vi "ACal-Update Probe Tube Parameters.vi"(0 "Params in":T1) -> (4 "Params out":T1)   [LabVIEW 2020]
uses:
  Type Defs/ACal-Probe Tube Parameters.ctl
  epl-vi-lib/Utility VIs/Type Defs/Left-Right ring.ctl
  Type Defs/Cal Stimulus.ctl
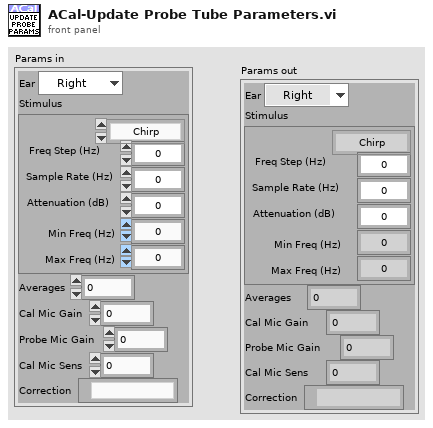
[diagram p1: front panel]
types:
  T1 = typedef "ACal-Probe Tube Parameters.ctl" = cluster{"Ear":T2, "Stimulus":T3, "Averages":i32, "Cal Mic Gain":dbl, "Probe Mic Gain":dbl, "Cal Mic Sens":dbl, "Correction":path}
  T2 = typedef "Left-Right ring.ctl" = enum16{"Right", "Left"}
  T3 = typedef "Cal Stimulus.ctl" = cluster{"Min Freq (Hz)":dbl, "Max Freq (Hz)":dbl, "Freq Step (Hz)":dbl, "Waveform":enum16{"Chirp", "Weighted"}, "Attenuation (dB)":dbl, "Sample Rate (Hz)":dbl}
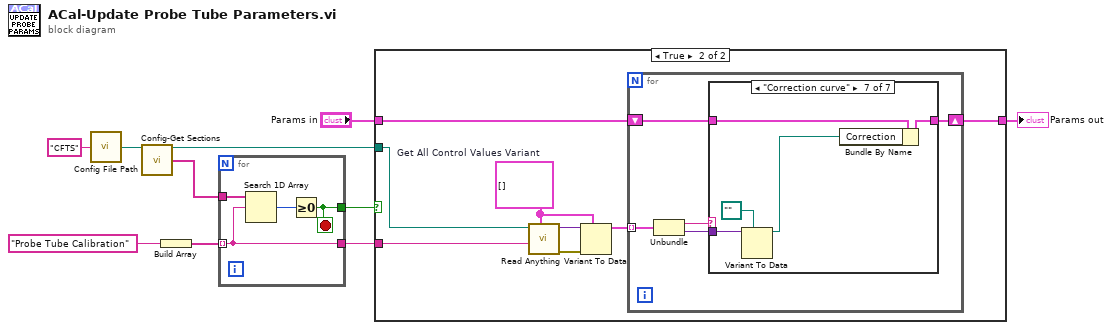
[diagram p0: block diagram]
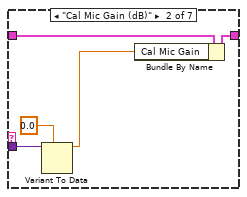
[diagram p4: hidden frame]
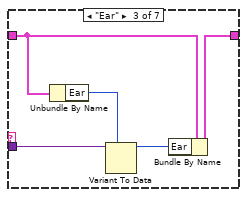
[diagram p5: hidden frame]
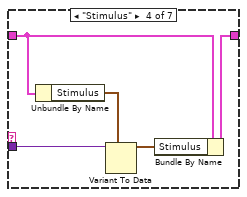
[diagram p6: hidden frame]
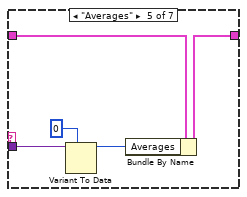
[diagram p7: hidden frame]
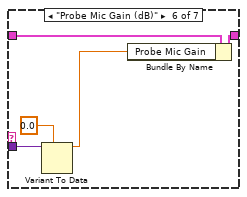
[diagram p8: hidden frame]
diagram:
  n1 = call "Config File Path.vi"("AppName"="CFTS") -> ("Default config file name"=w8:path)
  n2 = call "Config-Get Sections.vi"("configuration file path"=w8) -> ("file path"=w3:path, "section names"=w6:string[])  [unwired: 12 in, 1 out]
  n3 = Build Array("Probe Tube Calibration" ("element")) -> (w7:string[])
  n4 = for {
    tunnel: w7 -> [w11] mode=indexing
    tunnel: w6 -> [w14]
    tunnel: [w12] -> w5
    tunnel: [w11] -> w4
    stop <- w12 stop-if-true
    n5 = Search 1D Array(1D array=w14, element=w11) -> (index of element=w13:i32)  [unwired: 1 in]
    n6 = Greater Or Equal To 0?(x=w13) -> (x >= 0?=w12:bool)
  }
  n7 = case shown="True" w5 {
    tunnel: w4 -> [_ w23]
    tunnel: w3 -> [_ w22]
    tunnel: "Params in" -> [w15 w21]
    tunnel: [w15 w16] -> w1
    frame False {
    }
    frame True {
      w18 = cluster{"Name":string, "Variant Data":variant}[] []  # Get All Control Values Variant
      n8 = call "Read Anything.vi"("Type of Anything"=w18, "Section Name (Name of \"Type of Anything\")"=w23, "Path (dialog)"=w22) -> ("Error Out"=w20:errorcluster, "Anything"=w19:variant)  [unwired: 1 in, 6 out]
      n9 = Variant To Data(error in=w20, type=w18, Variant=w19) -> (data=w17:cluster{"Name":string, "Variant Data":variant}[])  [unwired: 1 out]
      n10 = for {
        shift-right: [w27] -> w16
        shift-left: w21 -> [w26]
        tunnel: w17 -> [w28] mode=indexing
        n11 = Unbundle(w28) -> ("Name"=w25:string, "Variant Data"=w24:variant)
        n12 = case shown="\"Correction curve\"" w25 {
          tunnel: [w29 w31 w38 w43 w48 w51 w56] -> w27
          tunnel: w26 -> [w29 w34 w36 w41 w46 w54 w59]
          tunnel: w24 -> [_ w33 w39 w44 w49 w53 w58]
          frame "", Default {
          }
          frame "Cal Mic Gain (dB)" {
            n13 = Variant To Data(type=0.0, Variant=w33) -> (data=w30:dbl)  [unwired: 1 in, 1 out]
            n14 = Bundle By Name(cluster=w34, "Cal Mic Gain"=w30) -> (w31:T1)
          }
          frame "Ear" {
            n15 = Unbundle By Name(w36) -> ("Ear"=w35:T2)
            n16 = Variant To Data(type=w35, Variant=w39) -> (data=w37:T2)  [unwired: 1 in, 1 out]
            n17 = Bundle By Name(cluster=w36, "Ear"=w37) -> (w38:T1)
          }
          frame "Stimulus" {
            n18 = Unbundle By Name(w41) -> ("Stimulus"=w40:T3)
            n19 = Variant To Data(type=w40, Variant=w44) -> (data=w42:T3)  [unwired: 1 in, 1 out]
            n20 = Bundle By Name(cluster=w41, "Stimulus"=w42) -> (w43:T1)
          }
          frame "Averages" {
            n21 = Variant To Data(type=0, Variant=w49) -> (data=w47:i32)  [unwired: 1 in, 1 out]
            n22 = Bundle By Name(cluster=w46, "Averages"=w47) -> (w48:T1)
          }
          frame "Probe Mic Gain (dB)" {
            n23 = Variant To Data(type=0.0, Variant=w53) -> (data=w50:dbl)  [unwired: 1 in, 1 out]
            n24 = Bundle By Name(cluster=w54, "Probe Mic Gain"=w50) -> (w51:T1)
          }
          frame "Correction curve" {
            n25 = Variant To Data(type=path "", Variant=w58) -> (data=w55:path)  [unwired: 1 in, 1 out]
            n26 = Bundle By Name(cluster=w59, "Correction"=w55) -> (w56:T1)
          }
        }
      }
    }
  }
  "Params out" <- w1
